vi "Message_ConvertClusterToClass.vi"(3 "OutputClusterType":cluster{"Numeric":dbl}, 11 "InputCluster":cluster{"Numeric":dbl}) -> (2 "OutputCluster":cluster{"Numeric":dbl})   [LabVIEW 2019, in "OneOfTemplate.lvclass"]
uses:
  OneOfTemplate.lvclass
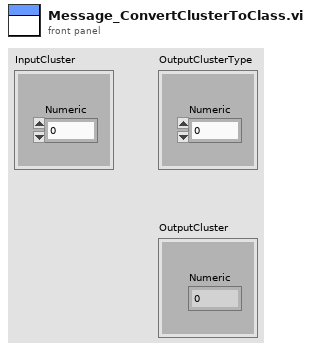
[diagram p1: front panel]
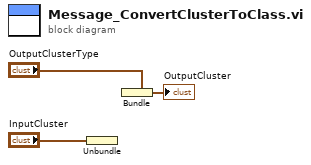
[diagram p0: block diagram]
diagram:
  n1 = Unbundle "Unbundle"("InputCluster") -> ()  [unwired: 1 out]
  n2 = Bundle "Bundle"(cluster="OutputClusterType") -> (→"OutputCluster":cluster{"Numeric":dbl})  [unwired: 1 in]
